vi "SR830_any.vi"(8 "error in (no error)":errorcluster, 10 "initial string":string="OFLT? ", 11 "VISA resource name":refnum<visa-resource-name>) -> (0 "error out":errorcluster, 2 "Measurement":dbl, 3 "VISA resource name out":refnum<visa-resource-name>)   [LabVIEW 2018]
doc: "Reads single parameter and returns single measurement from the instrument."
uses:
  <instrlib>/Stanford Research 830/Stanford Research 830.lvlib
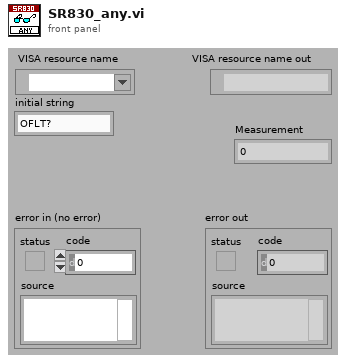
[diagram p1: front panel]
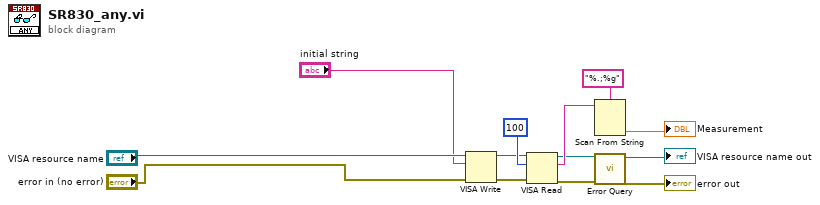
[diagram p0: block diagram]
diagram:
  n1 = VISA Write(VISA resource name="VISA resource name", write buffer="initial string", error in (no error)="error in (no error)") -> (VISA resource name out=w5:refnum<visa-resource-name>, error out=w4:errorcluster)  [unwired: 1 out]
  n2 = VISA Read(VISA resource name=w5, byte count=u32 100, error in (no error)=w4) -> (VISA resource name out=w7:refnum<visa-resource-name>, read buffer=w13:string, error out=w6:errorcluster)  [unwired: 1 out]
  n3 = Scan From String(format string="%.;%g", input string=w13) -> (output 1=→"Measurement":dbl)  [unwired: 3 in, 3 out]
  n4 = call <instrlib>:"Error Query.vi"("error in (no error)"=w6, "VISA resource name"=w7) -> ("error out"=→"error out":errorcluster, "VISA resource name out"=→"VISA resource name out":refnum<visa-resource-name>)  [unwired: 7 in, 1 out]
